vi "Format Sum of Asymmetric Gaussians Fit Parameters.vi"(8 "Step Size":dbl, 9 "R^2":dbl, 10 "MSE":dbl, 11 "Best Fit Parameters":dbl[](array[numeric])) -> (0 "# Components":i32, 3 "Array of Asymmetric Gaussian Fit Parameters":T1[](array[typedef]))   [LabVIEW 2021, in "Fits.lvlib"]
uses:
  Fits.lvlib
  Asymmetric Gaussian/Asymmetric Gaussian Fit Results v2.ctl
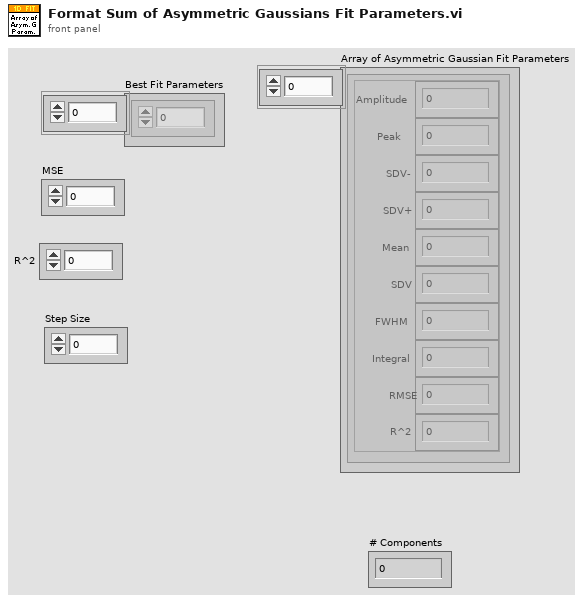
[diagram p1: front panel]
types:
  T1 = typedef "Fits.lvlib/Asymmetric Gaussian Fit Results v2.ctl" = cluster{"Amplitude":dbl, "Peak":dbl, "SDV-":dbl, "SDV+":dbl, "Mean":dbl, "SDV":dbl, "FWHM":dbl, "Integral":dbl, "RMSE":dbl, "R^2":dbl}
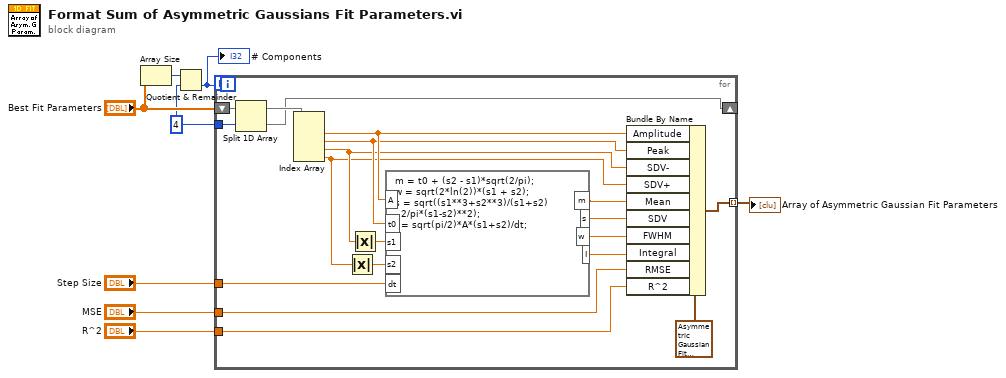
[diagram p0: block diagram]
diagram:
  w2 = 4 ("index")
  n1 = Array Size(array="Best Fit Parameters") -> (size(s)=w4:i32)
  n2 = Quotient & Remainder(x=w4, y=w2) -> (floor(x/y)=w3:i32)  [unwired: 1 out]
  "# Components" <- w3
  n3 = for {
    N: w3 -> [_]
    tunnel: "Step Size" -> [w26]
    tunnel: [w25] -> w6 mode=indexing
    tunnel: "MSE" -> [w10]
    shift-right: [w11] -> _
    shift-left: "Best Fit Parameters" -> [w27]
    tunnel: w2 -> [w13]
    tunnel: "R^2" -> [w9]
    n4 = Split 1D Array(array=w27, index=w13) -> (first subarray=w12:dbl[], second subarray=w11:dbl[])
    n5 = Index Array(array=w12) -> (element #1=w21:dbl, element #2=w20:dbl, element #3=w19:dbl, element #4=w18:dbl)  [unwired: 4 in]
    n6 = Absolute Value(x=w18) -> (abs(x)=w22:dbl)
    n7 = Absolute Value(x=w19) -> (abs(x)=w23:dbl)
    n8 = formula code="m = t0 + (s2 - s1)*sqrt(2/pi);\nw = sqrt(2*ln(2))*(s1 + s2);\ns = sqrt((s1**3+s2**3)/(s1+s2)\n- 2/pi*(s1-s2)**2);\nI = sqrt(pi/2)*A*(s1+s2)/dt;"("t0"=w20, "s1"=w23, "s2"=w22, "A"=w21, "dt"=w26) -> ("m"=w17:dbl, "w"=w15:dbl, "s"=w16:dbl, "I"=w14:dbl)
    n9 = Bundle By Name(cluster=T1 {"Amplitude"=0.0, "Peak"=0.0, "SDV-"=0.0, "SDV+"=0.0, "Mean"=0.0, "SDV"=0.0, "FWHM"=0.0, "Integral"=0.0, "RMSE"=0.0, "R^2"=0.0} ("Asymmetric Gaussian Fit Parameters"), "Amplitude"=w21, "Peak"=w20, "SDV-"=w19, "SDV+"=w18, "Mean"=w17, "SDV"=w16, "FWHM"=w15, "Integral"=w14, "RMSE"=w10, "R^2"=w9) -> (w25:T1)
  }
  "Array of Asymmetric Gaussian Fit Parameters" <- w6
